vi "Exit.vi"(8 "error in (no error)":errorcluster, 11 "Old State":refnum<class "Running Command.lvclass">) -> (0 "error out":errorcluster, 3 "New State":refnum<class "Running Command.lvclass">)   [LabVIEW 2014, in "Robot Actors.lvlib" / "Command Processor.lvlib" / "Running Command.lvclass"]
doc: "This is an abstract method. Override this method to define the behavior when you leave the state."
uses:
  Running Command.lvclass
  Command/Command Class/Command Status.ctl
  Command/Command Class/Command States.ctl
  <vilib>/ActorFramework/Message Enqueuer/Message Enqueuer.lvclass/Message Enqueuer.ctl
  <vilib>/ActorFramework/Message Enqueuer/Enqueue.vi
  <vilib>/ActorFramework/Message Priority Queue/Priority Enqueue.vi
  <vilib>/ActorFramework/Stop Msg/Stop Msg.lvclass
  Command Processor Class/Command Processor.lvclass
  Command/Command Class/Command.lvclass
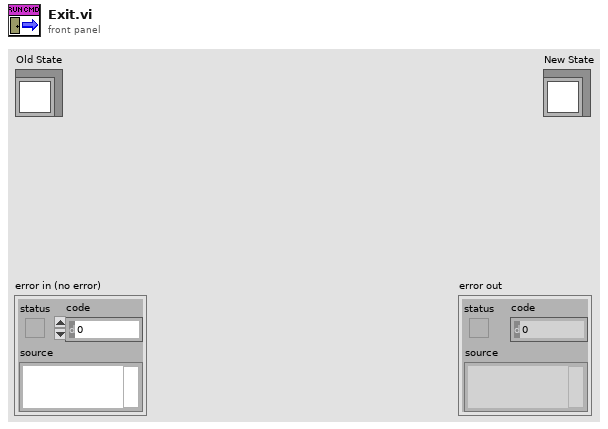
[diagram p1: front panel]
types:
  T1 = typedef "Robot Actors.lvlib/Command.lvlib/Command.lvclass/Command Status.ctl" = cluster{"Command Name":string, "Command Start Time":timestamp, "Command End Time":timestamp, "Is Command Finished?":bool, "Command ID":dbl, "Command State":T2}
  T2 = typedef "Robot Actors.lvlib/Command.lvlib/Command.lvclass/Command States.ctl" = enum16{"Unknown", "Started", "Stopped", "Finished"}
  T3 = typedef "Robot Actors.lvlib/Command Processor.lvlib/Command Processor.lvclass/Command Processor Status.ctl" = cluster{"Next Command ID":dbl, "Current Command Status":T1, "Previous Command Status ":T1, "Command Processor State":T4, "Last Status Update":timestamp}
  T4 = typedef "Robot Actors.lvlib/Command Processor.lvlib/Command Processor.lvclass/Command Processor States.ctl" = enum16{"Unknown", "No Command", "Running Command"}
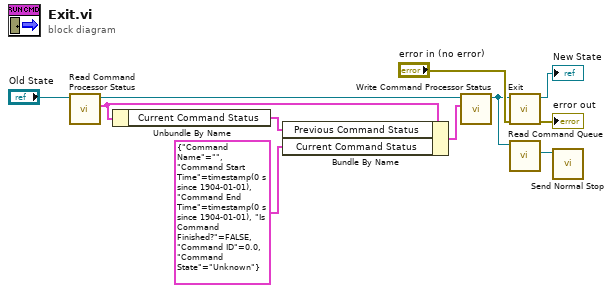
[diagram p0: block diagram]
diagram:
  n1 = call-dynamic "Read Command Processor Status.vi"("Command Processor in"="Old State") -> ("Command Processor Status"=w3:T3, "Command Processor out"=w5:refnum<class "Running Command.lvclass">)  [unwired: 8 in, 1 out]
  n2 = Unbundle By Name(w3) -> ("Current Command Status"=w2:T1)
  n3 = Bundle By Name(cluster=w3, "Previous Command Status"=w2, "Current Command Status"=T1 {"Command Name"="", "Command Start Time"=timestamp(0 s since 1904-01-01), "Command End Time"=timestamp(0 s since 1904-01-01), "Is Command Finished?"=FALSE, "Command ID"=0.0, "Command State"=enum."Unknown"}) -> (w4:T3)
  n4 = call-dynamic "Write Command Processor Status.vi"("Command Processor Status"=w4, "Command Processor in"=w5) -> ("Command Processor out"=w6:refnum<class "Running Command.lvclass">)  [unwired: 8 in, 1 out]
  n5 = call-parent "Exit.vi"("error in (no error)"="error in (no error)", "Old State"=w6) -> ("error out"=→"error out":errorcluster, "New State"=→"New State":refnum<class "Running Command.lvclass">)  [unwired: 8 in]
  n6 = call-dynamic "Read Command Queue.vi"("Command Processor in"=w6) -> ("Actor Framework:Message Enqueuer"=w8:refnum<class "Message Enqueuer.lvclass">)  [unwired: 8 in, 2 out]
  n7 = call <vilib>:"Send Normal Stop.vi"("Message Enqueuer"=w8) -> ()  [unwired: 10 in, 1 out]
